vi "LINC Insert Raw Data.vi"(5 "raw byte offset (0)":i32, 6 "sim ops":T2[](array[typedef]) {"mask" format="%02x"}, 7 "raw data":string, 8 "error in (no error)":errorcluster, 9 "data in":string, 10 "item formats in":T1[](array[typedef])) -> (0 "error out":errorcluster, 1 "data out":string)   [LabVIEW 2018, in "STEPkgDriver_LINC.lvlib"]
uses:
  STEPkgDriver_LINC.lvlib
  LINC Sim Ops.ctl
  LINC Format Prototype.ctl
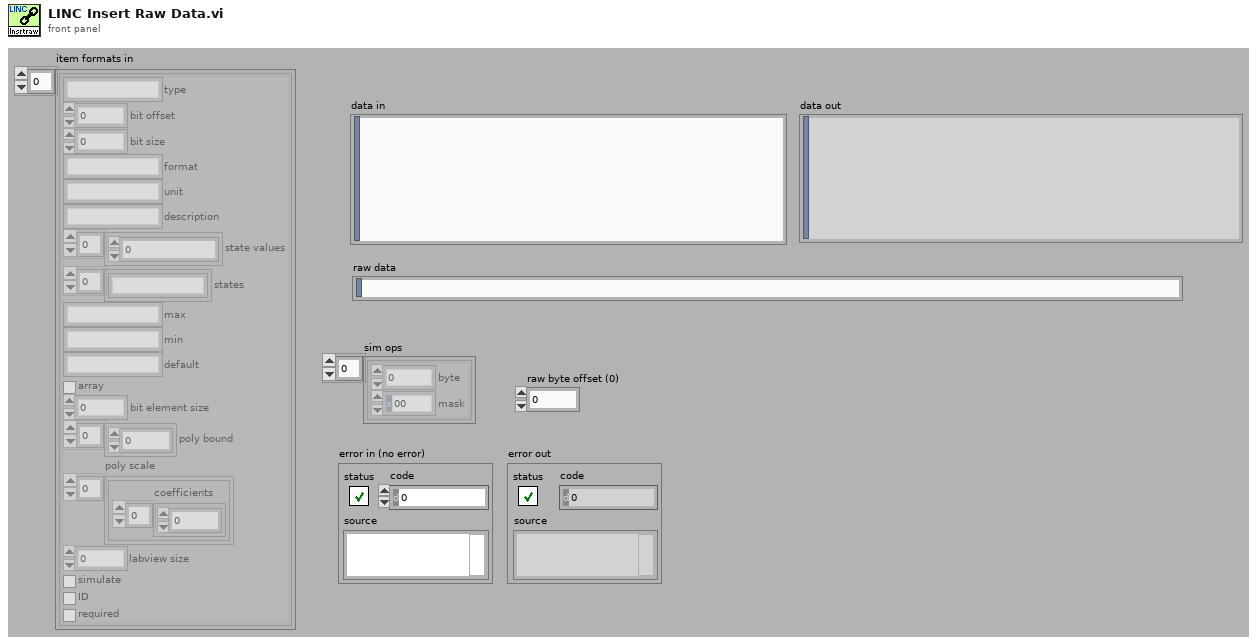
[diagram p1: front panel]
types:
  T1 = typedef "STEPkgDriver_LINC.lvlib/LINC Format Prototype.ctl" = cluster{"type":string, "bit offset":i32, "bit size":i32, "format":string, "unit":string, "description":string, "state values":i64[], "states":string[], "max":string, "min":string, "default":string, "array":bool, "bit element size":i32, "poly bound":dbl[], "poly scale":cluster{"coefficients":dbl[]}[], "labview size":i32, "simulate":bool, "ID":bool, "required":bool}
  T2 = typedef "STEPkgDriver_LINC.lvlib/LINC Sim Ops.ctl" = cluster{"byte":i32, "mask":u8}
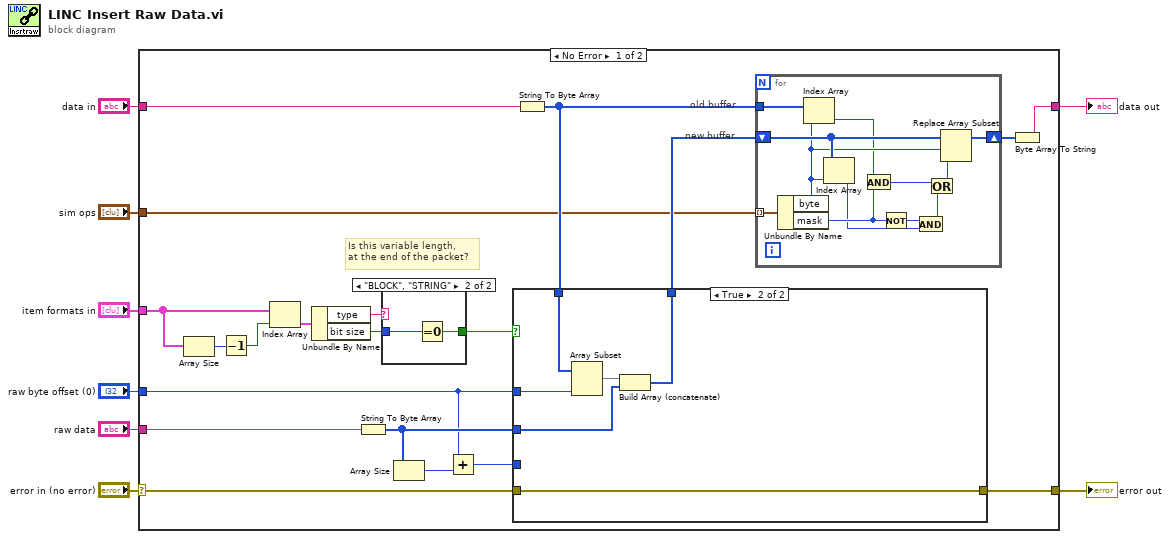
[diagram p0: block diagram]
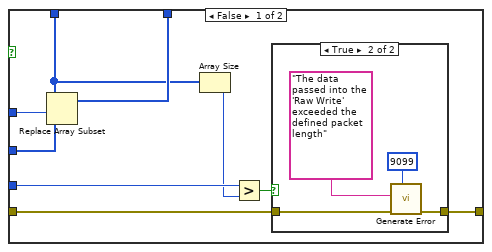
[diagram p3: hidden frame]
diagram:
  n1 = case shown="No Error" "error in (no error)" {
    selector: "error in (no error)" -> [w19 w63]
    tunnel: "data in" -> [w28 w64]
    tunnel: [w27 w64] -> w7
    tunnel: [w23 w63] -> w6
    tunnel: "raw byte offset (0)" -> [w18 _]
    tunnel: "raw data" -> [w17 _]
    tunnel: "item formats in" -> [w13 _]
    tunnel: "sim ops" -> [w9 _]
    frame No Error {
      # "Is this variable length,\nat the end of the packet?"
      # "new buffer"
      # "old buffer"
      n2 = Array Size(array=w13) -> (size(s)=w15:i32)
      n3 = Decrement(x=w15) -> (x-1=w14:i32)
      n4 = Index Array(array=w13, index=w14) -> (element=w10:T1)
      n5 = Unbundle By Name(w10) -> ("type"=w12:string, "bit size"=w11:i32)
      n6 = String To Byte Array(string=w17) -> (unsigned byte array=w26:u8[])
      n7 = case shown="\"BLOCK\", \"STRING\"" w12 {
        tunnel: w11 -> [_ w30]
        tunnel: [_ w29] -> w16
        frame Default {
        }
        frame "BLOCK", "STRING" {
          n8 = Equal To 0?(x=w30) -> (x = 0?=w29:bool)
        }
      }
      n9 = Array Size(array=w26) -> (size(s)=w25:i32)
      n10 = Add(x=w18, y=w25) -> (x+y=w24:i32)
      n11 = String To Byte Array(string=w28) -> (unsigned byte array=w20:u8[])
      n12 = case shown="True" w16 {
        tunnel: w26 -> [w38 w49]
        tunnel: w24 -> [w37 _]
        tunnel: [w35 w50] -> w23
        tunnel: [w34 w46] -> w22
        tunnel: w20 -> [w33 w48]
        tunnel: w19 -> [w32 w50]
        tunnel: w18 -> [w31 w47]
        frame False {
          n13 = Replace Array Subset(array=w33, new element=w38, index=w31) -> (w34:u8[])
          n14 = Array Size(array=w33) -> (size(s)=w36:i32)
          n15 = Greater?(x=w37, y=w36) -> (0:w39:bool)
          n16 = case shown="True" w39 {
            tunnel: w32 -> [w40 w42]
            tunnel: [w40 w41] -> w35
            frame False {
            }
            frame True {
              n17 = call "Generate Error.vi"("error code (-1301)"=9099, "error in"=w42, "description"="The data passed into the 'Raw Write' exceeded the defined packet length") -> ("error out"=w41:errorcluster)  [unwired: 8 in]
            }
          }
        }
        frame True {
          n18 = Array Subset(array=w48, length=w47) -> (w45:u8[])  [unwired: 1 in]
          n19 = Build Array (concatenate)(w45, w49) -> (w46:u8[])
        }
      }
      n20 = for {
        tunnel: w9 -> [w59] mode=indexing
        shift-right: [w56] -> w21
        shift-left: w22 -> [w57]
        tunnel: w20 -> [w58]
        n21 = Unbundle By Name(w59) -> ("byte"=w55:i32, "mask"=w53:u8)
        n22 = Index Array(array=w58, index=w55) -> (element=w54:u8)
        n23 = Index Array(array=w57, index=w55) -> (element=w52:u8)
        n24 = And(x=w54, y=w53) -> (x .and. y?=w62:u8)
        n25 = Not(x=w53) -> (.not. x?=w60:u8)
        n26 = And(x=w60, y=w52) -> (x .and. y?=w61:u8)
        n27 = Or(x=w62, y=w61) -> (x .or. y?=w51:u8)
        n28 = Replace Array Subset(array=w57, new element=w51, index=w55) -> (w56:u8[])
      }
      n29 = Byte Array To String(unsigned byte array=w21) -> (string=w27:string)
    }
    frame Error {
    }
  }
  "data out" <- w7
  "error out" <- w6
